vi "main.vi"() -> ()   [LabVIEW 2019]
uses:
  Controls/50cents.ctl
  Controls/20cents.ctl
  Controls/10cents.ctl
  Controls/data.ctl
  Controls/states.ctl
panel:
  out "Deposited":string
  in  "10cents":T1
  in  "20cents":T2
  in  "50cents":T3
  out "Pict Ring":u16(ring)
  in  "Stop Button":bool
  out "Current State":string
  out "Change Return":string
  in  "Return Money":bool
  in  "Orange":bool
  in  "Apple":bool
  in  "Lemond":bool
  # "90 Cents"
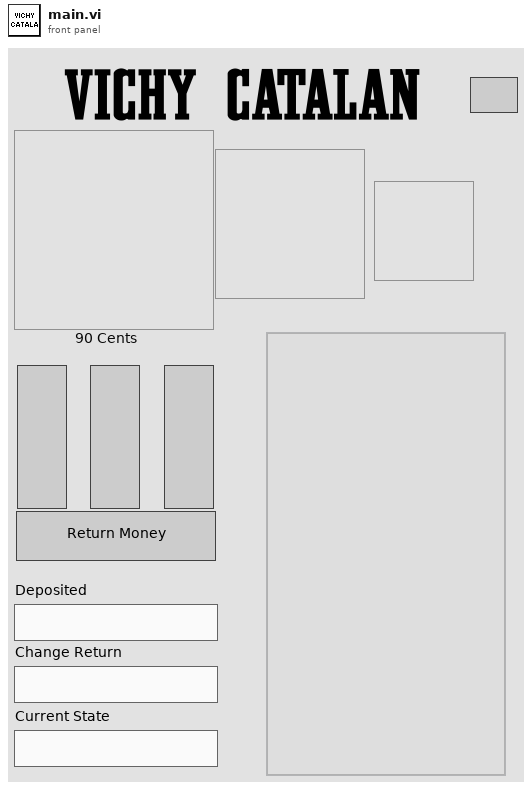
[diagram p1: front panel]
types:
  T1 = typedef "10cents.ctl" = bool
  T2 = typedef "20cents.ctl" = bool
  T3 = typedef "50cents.ctl" = bool
  T4 = typedef "states.ctl" = enum16{"Initialize", "Wait for Event", "50cents", "20cents", "10cents", "Lemond", "Apple", "Orange", "Return Money", "Delivery", "Exit"}
  T5 = typedef "data.ctl" = cluster{"Deposited":dbl, "Choosen":bool}
  T6 = enum8{"Enabled", "Disabled", "Disabled and Grayed Out"}
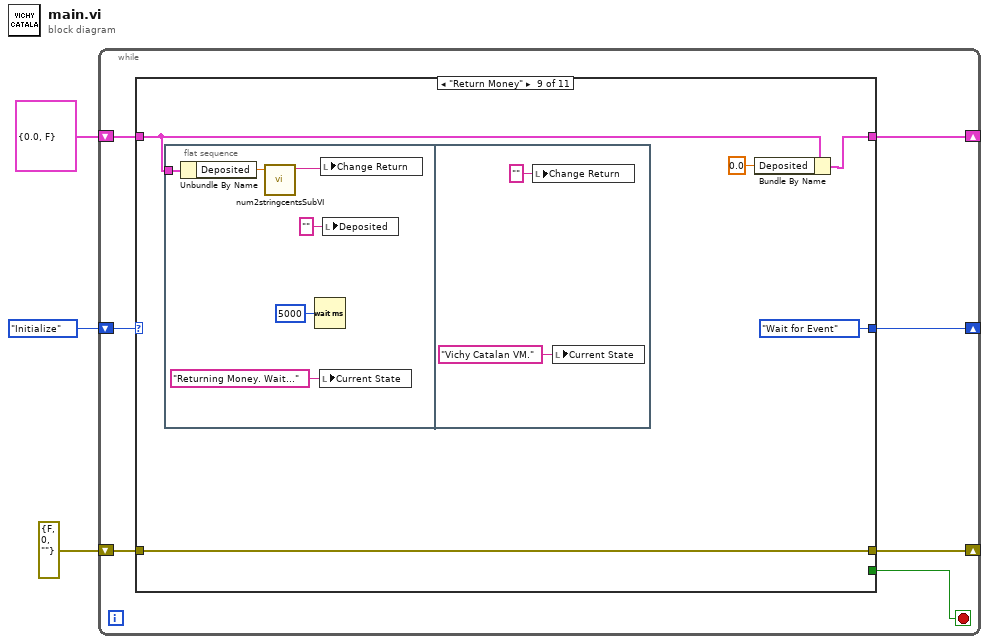
[diagram p0: block diagram]
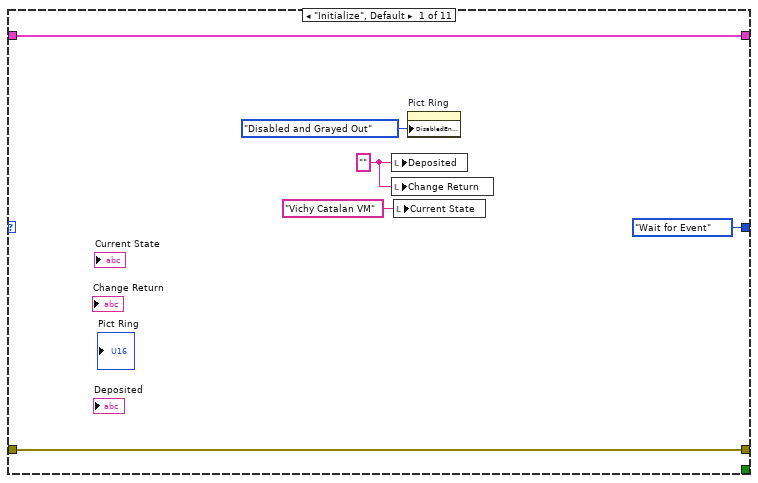
[diagram p2: hidden frame]
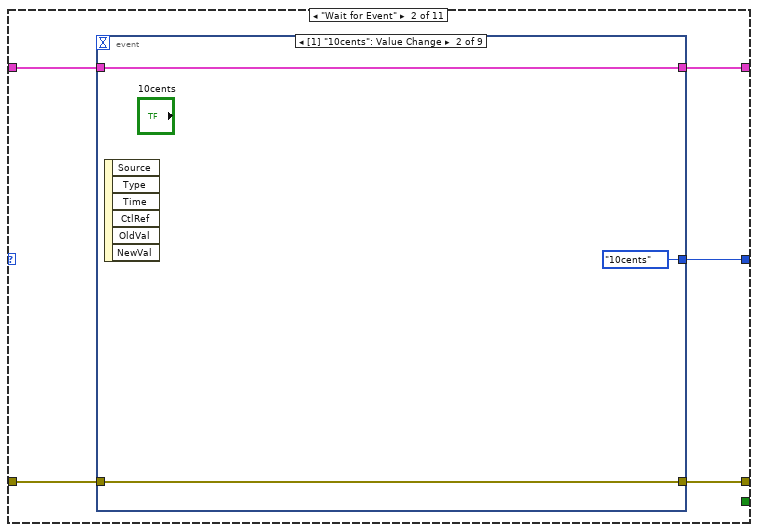
[diagram p3: hidden frame]
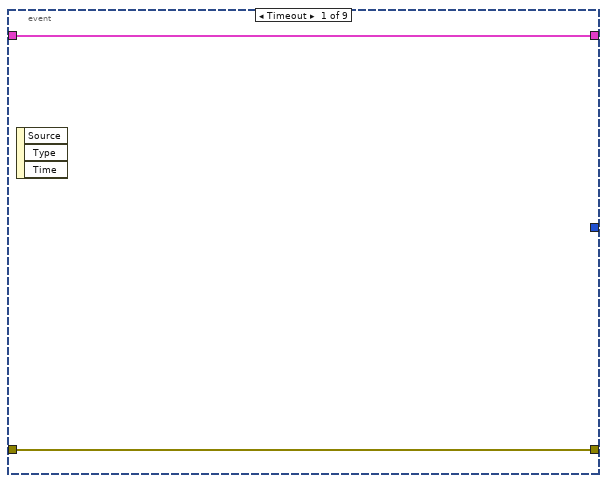
[diagram p4: hidden frame]
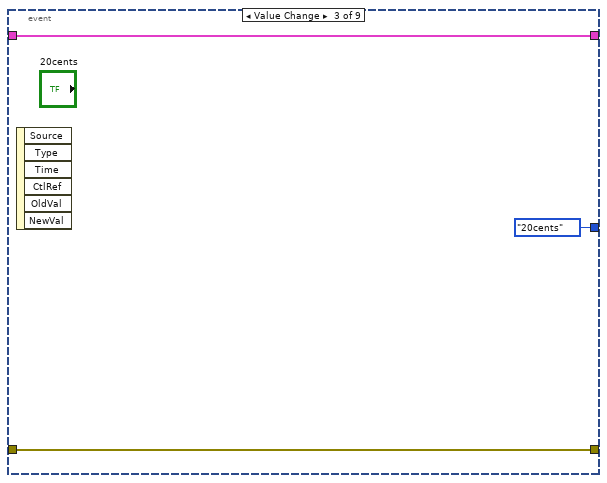
[diagram p5: hidden frame]
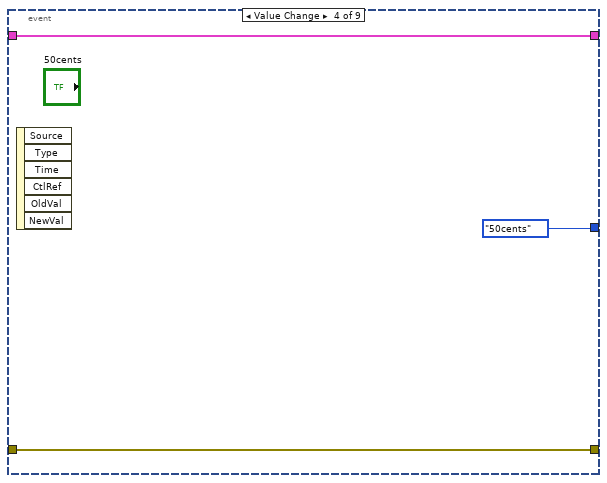
[diagram p6: hidden frame]
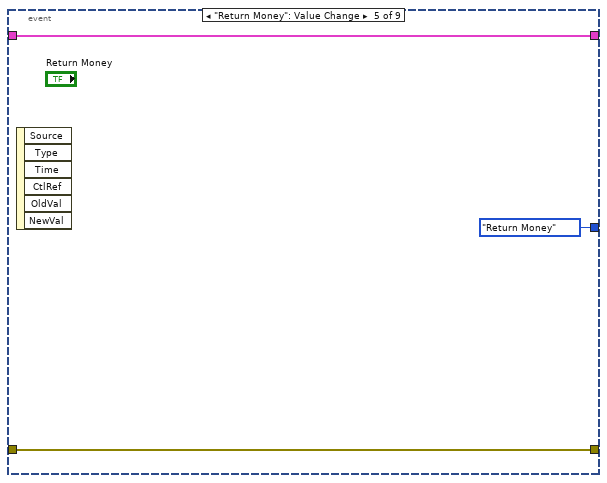
[diagram p7: hidden frame]
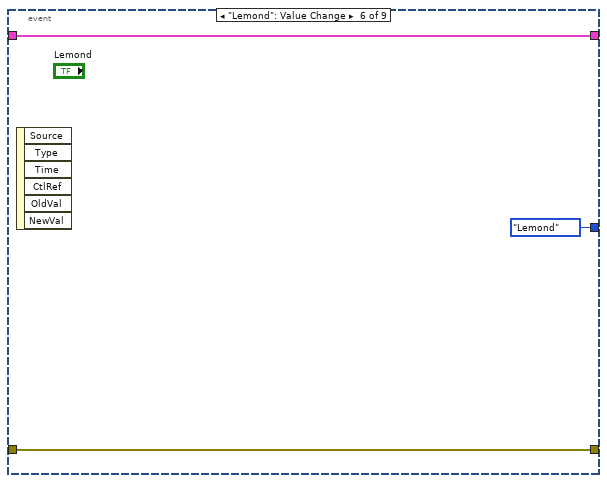
[diagram p8: hidden frame]
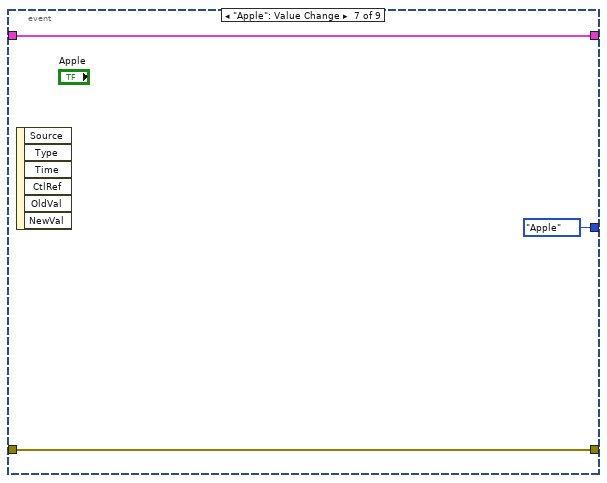
[diagram p9: hidden frame]
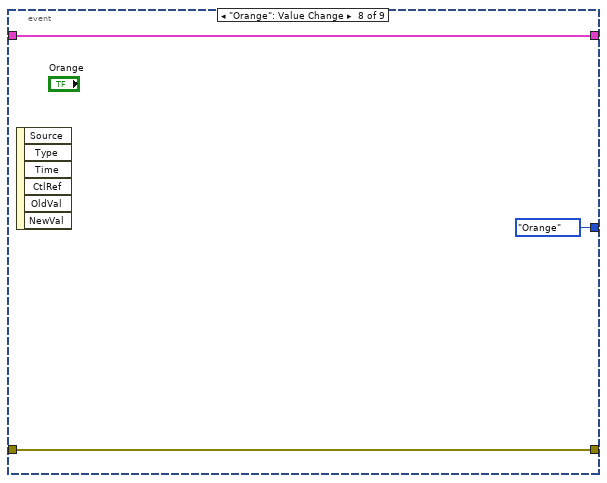
[diagram p10: hidden frame]
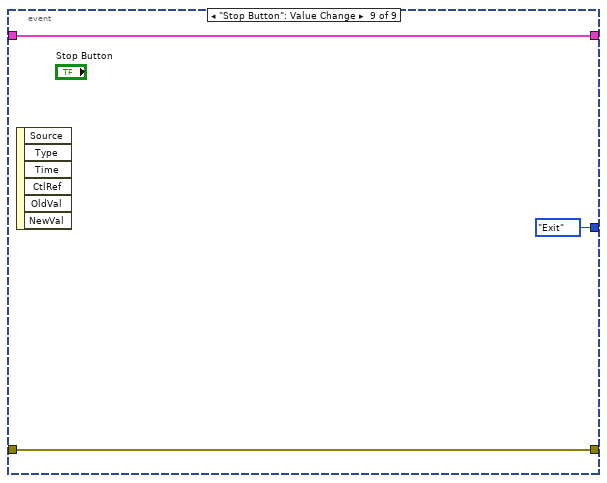
[diagram p11: hidden frame]
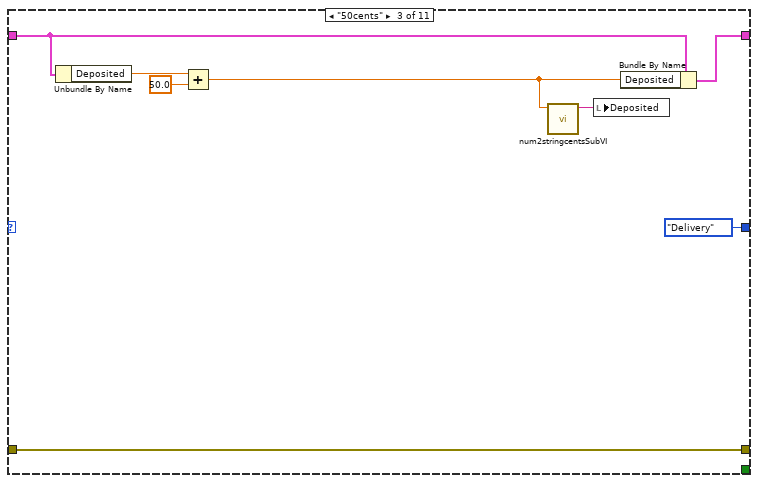
[diagram p12: hidden frame]
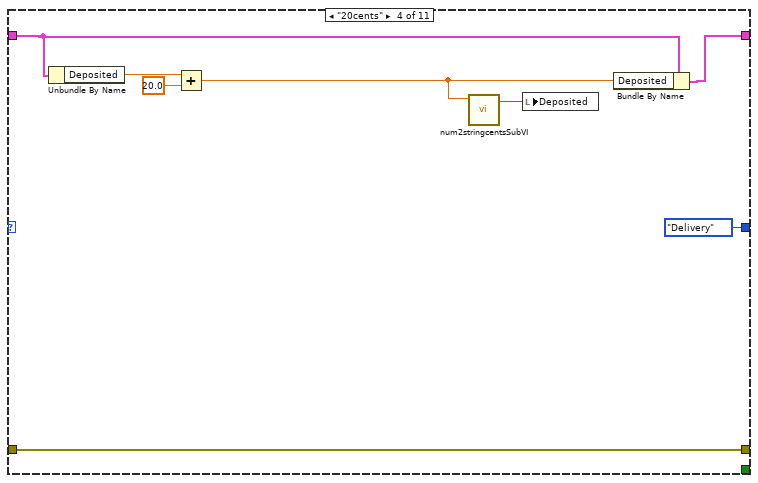
[diagram p13: hidden frame]
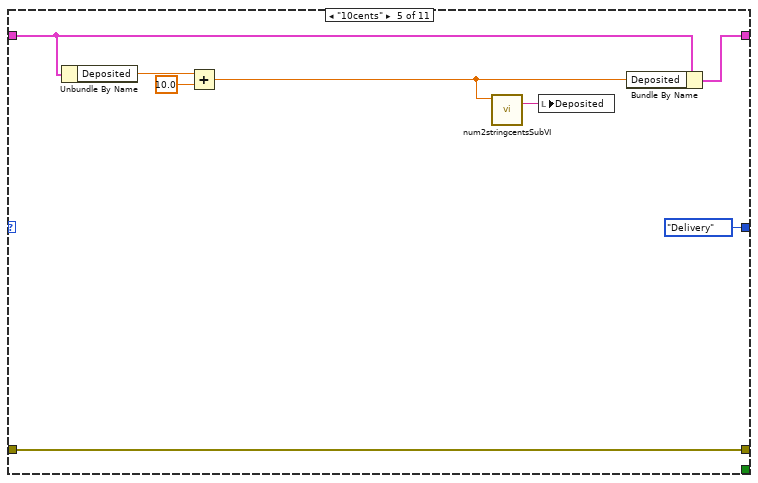
[diagram p14: hidden frame]
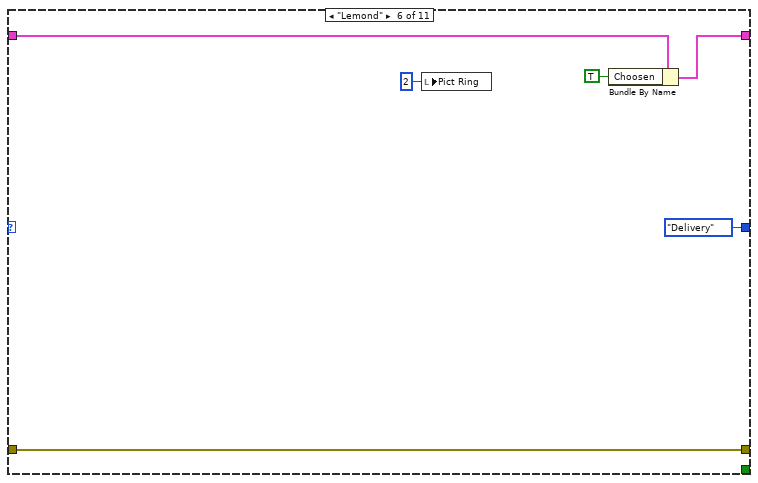
[diagram p15: hidden frame]
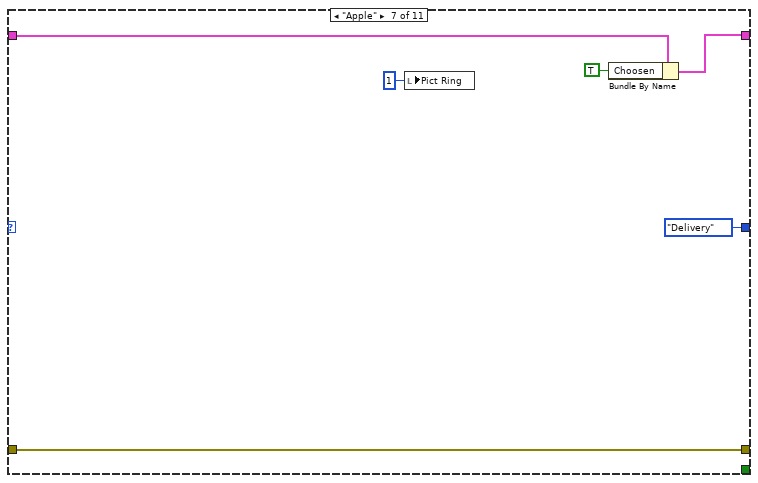
[diagram p16: hidden frame]
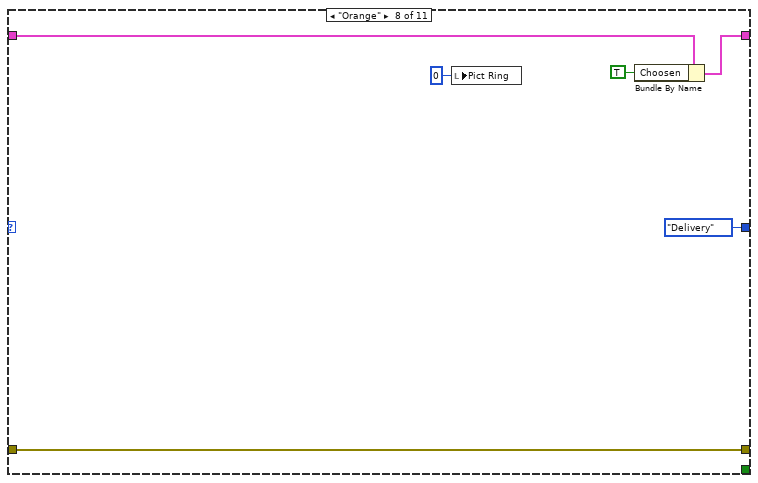
[diagram p17: hidden frame]
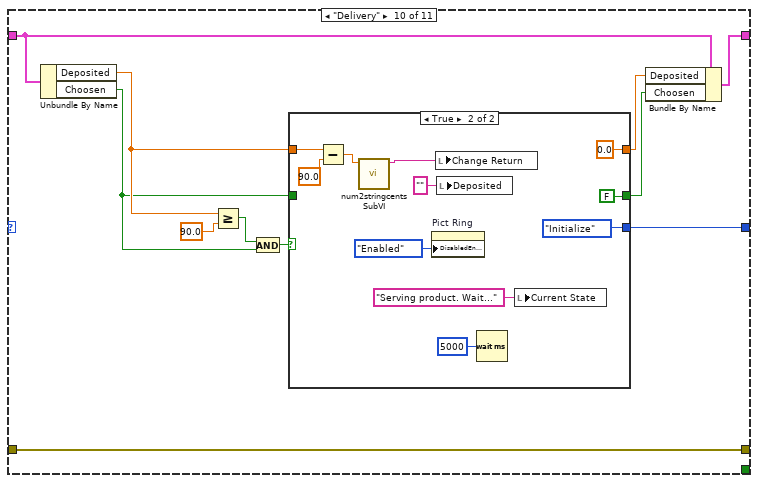
[diagram p18: hidden frame]
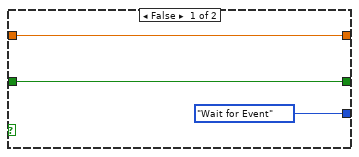
[diagram p19: hidden frame]
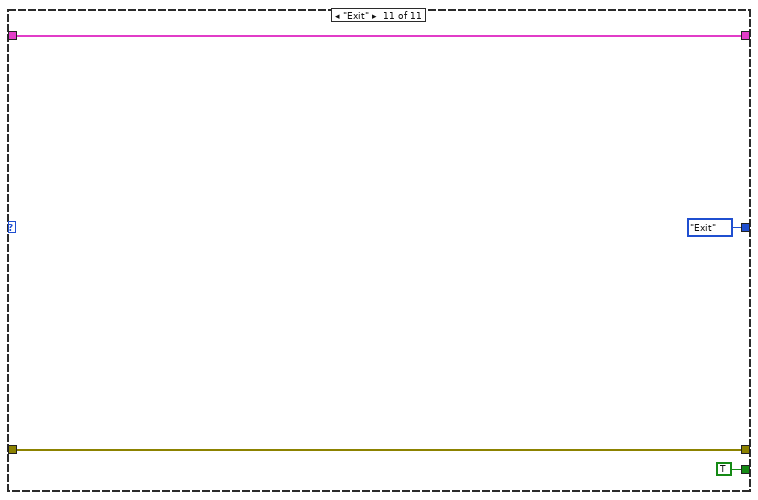
[diagram p20: hidden frame]
diagram:
  n1 = while {
    shift-right: [w7] -> _
    shift-left: states."Initialize" ("Enum") -> [w10]
    shift-right: [w4] -> _
    shift-left: T5 {"Deposited"=0.0, "Choosen"=FALSE} ("Cluster") -> [w6]
    shift-right: [w8] -> _
    shift-left: errorcluster {"status"=FALSE, "code"=0, "source"=""} ("error constant") -> [w9]
    stop <- w5 stop-if-true
    n2 = case shown="\"Return Money\"" w10 {
      tunnel: w9 -> [w16 w21 w54 w62 w70 w76 w82 w88 w93 w113 w129]
      tunnel: [w16 w20 w54 w62 w70 w76 w82 w88 w93 w113 w129] -> w8
      tunnel: [states."Wait for Event" ("Enum") w17 states."Delivery" ("Enum") states."Delivery" ("Enum") states."Delivery" ("Enum") states."Delivery" ("Enum") states."Delivery" ("Enum") states."Delivery" ("Enum") states."Wait for Event" ("Enum") w107 states."Exit" ("Enum")] -> w7
      tunnel: w6 -> [w14 w19 w53 w57 w65 w75 w81 w87 w92 w109 w130]
      tunnel: [w14 w18 w50 w56 w64 w73 w80 w86 w91 w110 w130] -> w4
      tunnel: [_ _ _ _ _ _ _ _ _ _ TRUE] -> w5
      frame "Initialize", Default {
        w11 = "" ("Deposited")
        n3 = local write "Deposited"(w11) -> ()
        n4 = local write "Change Return"(w11) -> ()
        n5 = local write "Current State"("Vichy Catalan VM" ("Cureent State")) -> ()
        n6 = property on="Pict Ring" class="Ring (strict)"("DisabledEnum"=T6."Disabled and Grayed Out" ("Disabled")) -> ()  [unwired: 2 in, 2 out]
      }
      frame "Wait for Event" {
        n7 = event shown="[1] \"10cents\": Value Change" {
          selector: _ -> [_ _ _ _ _ _ _ _ _]
          dyn-events: _ -> [_ _ _ _ _ _ _ _ _]
          timeout: _ -> [_ _ _ _ _ _ _ _ _]
          tunnel: w21 -> [w23 w24 w27 w30 w33 w36 w39 w42 w45]
          tunnel: [w23 w24 w27 w30 w33 w36 w39 w42 w45] -> w20
          tunnel: [w22 w25 w28 w31 w34 w37 w40 w43 w46] -> w18
          tunnel: w19 -> [w22 w25 w28 w31 w34 w37 w40 w43 w46]
          tunnel: [_ states."10cents" ("Enum") states."20cents" ("Enum") states."50cents" ("Enum") states."Return Money" ("Enum") states."Lemond" ("Enum") states."Apple" ("Enum") states."Orange" ("Enum") states."Exit" ("Enum")] -> w17
          event Timeout {
            n8 = event-data() -> ()  [unwired: 1 in, 3 out]
          }
          event Value Change {
            n9 = event-data() -> ()  [unwired: 1 in, 6 out]
          }
          event Value Change {
            n10 = event-data() -> ()  [unwired: 1 in, 6 out]
          }
          event Value Change {
            n11 = event-data() -> ()  [unwired: 1 in, 6 out]
          }
          event "Return Money": Value Change {
            n12 = event-data() -> ()  [unwired: 1 in, 6 out]
          }
          event "Lemond": Value Change {
            n13 = event-data() -> ()  [unwired: 1 in, 6 out]
          }
          event "Apple": Value Change {
            n14 = event-data() -> ()  [unwired: 1 in, 6 out]
          }
          event "Orange": Value Change {
            n15 = event-data() -> ()  [unwired: 1 in, 6 out]
          }
          event "Stop Button": Value Change {
            n16 = event-data() -> ()  [unwired: 1 in, 6 out]
          }
        }
      }
      frame "50cents" {
        n17 = Unbundle By Name(w53) -> ("Deposited"=w52:dbl)
        n18 = Add(x=w52, y=50.0) -> (x+y=w48:dbl)
        n19 = call "num2stringcentsSubVI.vi"("Num"=w48) -> ("String with cents"=w49:string)  [unwired: 10 in]
        n20 = local write "Deposited"(w49) -> ()
        n21 = Bundle By Name(cluster=w53, "Deposited"=w48) -> (w50:T5)
      }
      frame "20cents" {
        n22 = Unbundle By Name(w57) -> ("Deposited"=w61:dbl)
        n23 = Add(x=w61, y=20.0) -> (x+y=w58:dbl)
        n24 = call "num2stringcentsSubVI.vi"("Num"=w58) -> ("String with cents"=w59:string)  [unwired: 10 in]
        n25 = local write "Deposited"(w59) -> ()
        n26 = Bundle By Name(cluster=w57, "Deposited"=w58) -> (w56:T5)
      }
      frame "10cents" {
        n27 = Unbundle By Name(w65) -> ("Deposited"=w69:dbl)
        n28 = Add(x=w69, y=10.0) -> (x+y=w67:dbl)
        n29 = call "num2stringcentsSubVI.vi"("Num"=w67) -> ("String with cents"=w66:string)  [unwired: 10 in]
        n30 = local write "Deposited"(w66) -> ()
        n31 = Bundle By Name(cluster=w65, "Deposited"=w67) -> (w64:T5)
      }
      frame "Lemond" {
        n32 = local write "Pict Ring"(u16 2 ("Pict Ring")) -> ()
        n33 = Bundle By Name(cluster=w75, "Choosen"=TRUE) -> (w73:T5)
      }
      frame "Apple" {
        n34 = local write "Pict Ring"(u16 1 ("Pict Ring")) -> ()
        n35 = Bundle By Name(cluster=w81, "Choosen"=TRUE) -> (w80:T5)
      }
      frame "Orange" {
        n36 = local write "Pict Ring"(u16 0 ("Pict Ring")) -> ()
        n37 = Bundle By Name(cluster=w87, "Choosen"=TRUE) -> (w86:T5)
      }
      frame "Return Money" {
        n38 = flat-sequence {
          tunnel: w92 -> [w100]
          frame #0 {
            n39 = Unbundle By Name(w100) -> ("Deposited"=w99:dbl)
            n40 = call "num2stringcentsSubVI.vi"("Num"=w99) -> ("String with cents"=w97:string)  [unwired: 10 in]
            n41 = Wait (ms)(milliseconds to wait=u32 5000) -> ()  [unwired: 1 out]
            n42 = local write "Current State"("Returning Money. Wait..." ("Cureent State")) -> ()
            n43 = local write "Change Return"(w97) -> ()
            n44 = local write "Deposited"("" ("Deposited")) -> ()
          }
          frame #1 {
            n45 = local write "Change Return"("" ("Change Return")) -> ()
            n46 = local write "Current State"("Vichy Catalan VM." ("Cureent State")) -> ()
          }
        }
        n47 = Bundle By Name(cluster=w92, "Deposited"=0.0) -> (w91:T5)
      }
      frame "Delivery" {
        n48 = Unbundle By Name(w109) -> ("Deposited"=w106:dbl, "Choosen"=w103:bool)
        n49 = Greater Or Equal?(x=w106, y=90.0) -> (x >= y?=w111:bool)
        n50 = And(x=w111, y=w103) -> (x .and. y?=w108:bool)
        n51 = case shown="True" w108 {
          tunnel: [states."Wait for Event" ("Enum") states."Initialize" ("Enum")] -> w107
          tunnel: w106 -> [w115 w119]
          tunnel: [w115 0.0 ("Deposited")] -> w105
          tunnel: [w114 FALSE] -> w104
          tunnel: w103 -> [w114 _]
          frame False {
          }
          frame True {
            n52 = Subtract(x=w119, y=90.0) -> (x-y=w117:dbl)
            n53 = call "num2stringcentsSubVI.vi"("Num"=w117) -> ("String with cents"=w122:string)  [unwired: 10 in]
            n54 = property on="Pict Ring" class="Ring (strict)"("DisabledEnum"=T6."Enabled" ("Disabled")) -> ()  [unwired: 2 in, 2 out]
            n55 = local write "Change Return"(w122) -> ()
            n56 = local write "Deposited"("" ("Deposited")) -> ()
            n57 = Wait (ms)(milliseconds to wait=u32 5000) -> ()  [unwired: 1 out]
            n58 = local write "Current State"("Serving product. Wait..." ("Cureent State")) -> ()
          }
        }
        n59 = Bundle By Name(cluster=w109, "Deposited"=w105, "Choosen"=w104) -> (w110:T5)
      }
      frame "Exit" {
      }
    }
  }
